vi "AutoDriveCheckDone.vi"(6 "Finished":bool caption="Auto distance Finished", 9 "DriveMinTime":u32, 10 "DriveTimeout":u32, 11 "millisecond timer value":u32) -> (1 "Boolean":bool, 2 "Stop?":bool, 3 "Timed out?":bool)   [LabVIEW 2013]
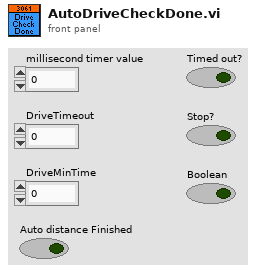
[diagram p1: front panel]
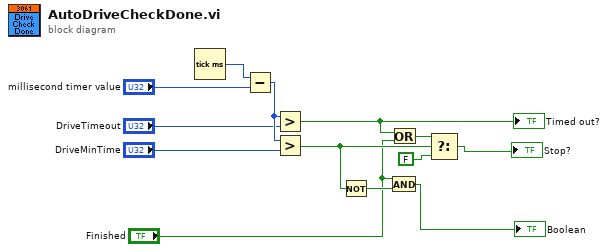
[diagram p0: block diagram]
diagram:
  n1 = Tick Count (ms)() -> (millisecond timer value=w1:u32)
  n2 = Subtract(x=w1, y="millisecond timer value") -> (x-y=w4:u32)
  n3 = Greater?(x=w4, y="DriveTimeout") -> (0:w6:bool)
  "Timed out?" <- w6
  n4 = Greater?(x=w4, y="DriveMinTime") -> (0:w11:bool)
  n5 = Not(x=w11) -> (.not. x?=w12:bool)
  n6 = And(x="Finished", y=w12) -> (x .and. y?=→"Boolean":bool)
  n7 = Or(x=w6, y="Finished") -> (x .or. y?=w7:bool)
  n8 = Select(t=w7, s=w11, f=FALSE) -> (s? t:f=→"Stop?":bool)
